vi "newsubvi Robot Index to Zero.vi"(0 "VISA In":refnum<visa-resource-name>) -> (1 "VISA Out":refnum<visa-resource-name>, 2 "Success":bool)   [LabVIEW 2012]
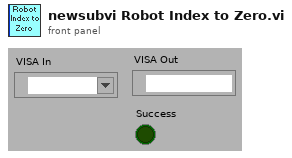
[diagram p1: front panel]
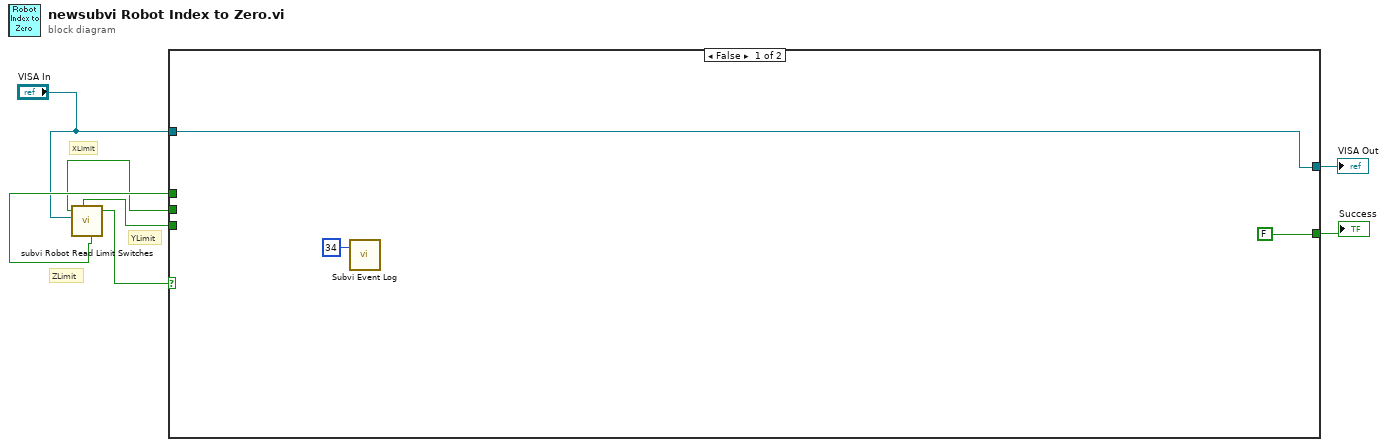
[diagram p0: block diagram]
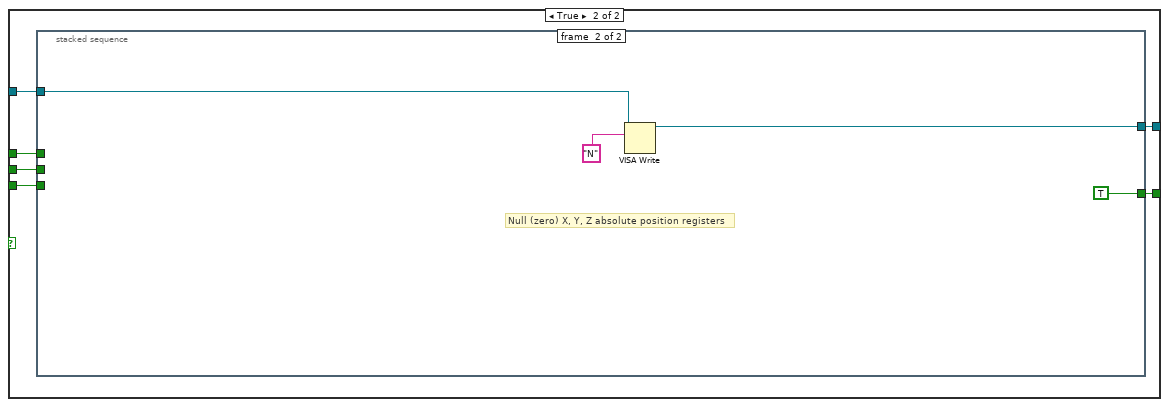
[diagram p2: hidden frame]
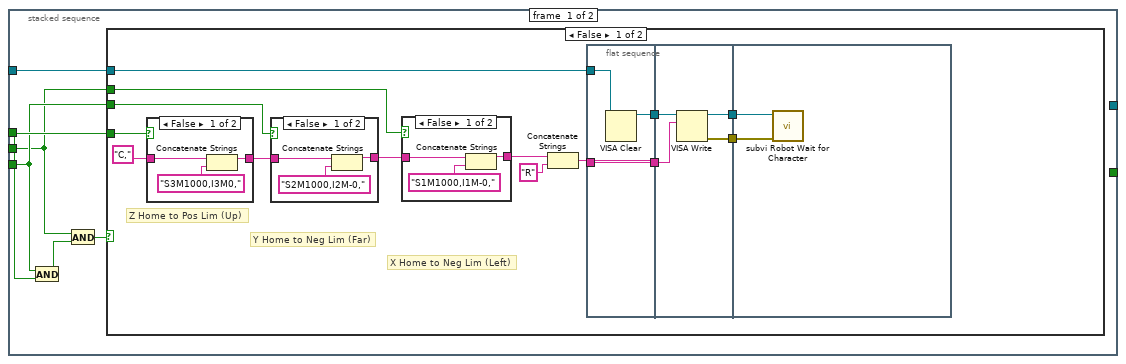
[diagram p3: hidden frame]
diagram:
  # "YLimit"
  # "XLimit"
  # "ZLimit"
  n1 = call "subvi Robot Read Limit Switches.vi"("VISA In"="VISA In") -> ("M1NegLim"=w5:bool, "M2NegLim"=w6:bool, "ReadOK"=w3:bool, "M3PosLim"=w7:bool)  [unwired: 5 out]
  n2 = case shown="False" w3 {
    tunnel: w7 -> [_ w16]
    tunnel: w6 -> [_ w15]
    tunnel: w5 -> [_ w14]
    tunnel: "VISA In" -> [w10 w13]
    tunnel: [w10 w12] -> w4
    tunnel: [FALSE w11] -> w2
    frame False {
      n3 = call "Subvi Event Log.vi"("EventNum"=u32 34) -> ()  [unwired: 1 in]
    }
    frame True {
      n4 = stacked-sequence {
        tunnel: w16 -> [w22 _]
        tunnel: w15 -> [w21 _]
        tunnel: w14 -> [w20 _]
        tunnel: w13 -> [w17 w61]
        tunnel: [_ w59] -> w12
        tunnel: [_ TRUE] -> w11
        frame #0 {
          n5 = And(x=w21, y=w22) -> (x .and. y?=w19:bool)
          n6 = And(x=w20, y=w19) -> (x .and. y?=w18:bool)
          n7 = case shown="False" w18 {
            tunnel: w22 -> [w30 _]
            tunnel: w21 -> [w29 _]
            tunnel: w20 -> [w28 _]
            tunnel: w17 -> [w26 _]
            frame False {
              # "X Home to Neg Lim (Left)"
              # "Y Home to Neg Lim (Far)"
              # "Z Home to Pos Lim (Up)"
              n8 = case shown="False" w30 {
                tunnel: "C," ("Text to Send") -> [w56 w57]
                tunnel: [w54 w57] -> w34
                frame False {
                  n9 = Concatenate Strings(w56, "S3M1000,I3M0," ("Text to Send")) -> (w54:string)
                }
                frame True {
                }
              }
              n10 = case shown="False" w29 {
                tunnel: w34 -> [w52 w53]
                tunnel: [w50 w53] -> w33
                frame False {
                  n11 = Concatenate Strings(w52, "S2M1000,I2M-0," ("Text to Send")) -> (w50:string)
                }
                frame True {
                }
              }
              n12 = case shown="False" w28 {
                tunnel: w33 -> [w48 w49]
                tunnel: [w46 w49] -> w32
                frame False {
                  n13 = Concatenate Strings(w48, "S1M1000,I1M-0," ("Text to Send")) -> (w46:string)
                }
                frame True {
                }
              }
              n14 = Concatenate Strings(w32, "R" ("string")) -> (w27:string)
              n15 = flat-sequence {
                tunnel: w27 -> [w39]
                tunnel: [w39] -> w36
                tunnel: w26 -> [w38]
                tunnel: [w37] -> w25
                tunnel: w36 -> [w42]
                tunnel: w25 -> [w43]
                tunnel: [w41] -> w24
                tunnel: [w40] -> w23
                tunnel: w24 -> [w45]
                tunnel: w23 -> [w44]
                frame #0 {
                  n16 = VISA Clear(VISA resource name=w38) -> (VISA resource name out=w37:refnum<visa-resource-name>)  [unwired: 1 in, 1 out]
                }
                frame #1 {
                  n17 = VISA Write(VISA resource name=w43, write buffer=w42) -> (VISA resource name out=w41:refnum<visa-resource-name>, error out=w40:errorcluster)  [unwired: 1 in, 1 out]
                }
                frame #2 {
                  n18 = call "subvi Robot Wait for Character.vi"("error in"=w44, "VISA In"=w45) -> ()  [unwired: 2 out]
                }
              }
            }
            frame True {
              # "All Limit Switches are ON\nDon't do anything\nIndex to Zero in next Sequence"
            }
          }
        }
        frame #1 {
          # "Null (zero) X, Y, Z absolute position registers"
          n19 = VISA Write(VISA resource name=w61, write buffer="N" ("Text to Send")) -> (VISA resource name out=w59:refnum<visa-resource-name>)  [unwired: 1 in, 2 out]
        }
      }
    }
  }
  "VISA Out" <- w4
  "Success" <- w2
